vi "get Camera Data LV.vi"(8 "error in (no error)":errorcluster, 11 "dataIn":u32[](array[numeric])) -> (0 "error out":errorcluster, 3 "dataOut":u32[](array[numeric]))   [LabVIEW 2016, in "cameraLibrary.lvlib"]
doc: "Returns the camera data in the provided array.\n\n\n\nvoid CAMERALIBRARYSHARED_EXPORT getCameraDataLV(long *dataOut);"
uses:
  cameraLibrary.lvlib
  cameraLibrary.dll
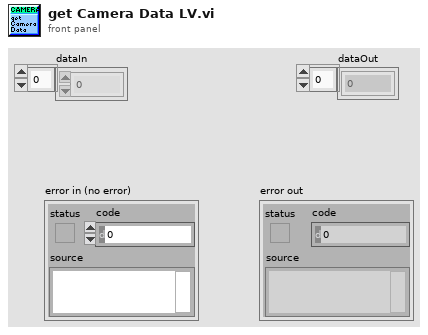
[diagram p1: front panel]
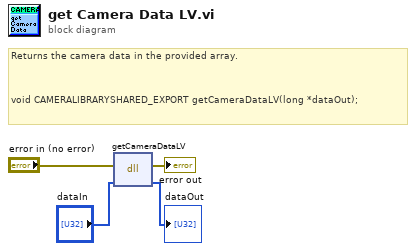
[diagram p0: block diagram]
diagram:
  # "Returns the camera data in the provided array.\n\n\n\nvoid CAMERALIBRARYSHARED_EXPORT getCameraDataLV(long *dataOut);"
  n1 = dll-call lib="C:/Users/TMM/repos/EXPRES/FEM/FTT/support/Camera Library/cameraLibrary.*" fn="getCameraDataLV"(error in="error in (no error)", "dataOut"="dataIn") -> (error out=→"error out":errorcluster, "dataOut"=→"dataOut":u32[])  [unwired: 3 in, 1 out]
